vi "MF-101 Analog Output with diags and disk file.vi"() -> ()   [LabVIEW 8.6]
uses:
  <libdir>/resource/objmgr/ueidaq.rc
  <vilib>/Utility/file.llb/Write Delimited Spreadsheet (string).vi
  vi.lib/UeiDaq/UeiDaqConfigureTimingForSimpleIO.vi
  <vilib>/Utility/file.llb/Write Delimited Spreadsheet (DBL).vi
  vi.lib/UeiDaq/UeiDaqWriteOneScaledScan.vi
  vi.lib/UeiDaq/UeiDaqCreateAOSession.vi
  vi.lib/UeiDaq/UeiDaqCreateAOCurrentSession.vi
  vi.lib/UeiDaq/UeiDaqReadOneScaledScan.vi
panel:
  out "Diag Data":dbl[](array[numeric])
  in  "Diagnostic Resource":string
  in  "Maximum range":dbl
  in  "Minimum range":dbl
  in  "analog output":bool
  out "data points":i32
  in  "delta output":dbl format="%#_6f"
  in  "end  output":dbl
  in  "start output":dbl
  out "serial number":string
  out "name":string
  out "Waveform Chart":T1(graph)
  out "analog output(s)":dbl[](array[numeric])
  out "amplitude":dbl format="%#.6f"
  in  "Refresh rate (ms)":u32
  in  "stop":bool
  in  "Resource":string
  # "MF-101 Analog Output with Guardian diagnostics and disk file"
  # "Resource"
  # "Analog output settings"
  # "Device information"
  # "volts"
  # "amps"
  # "Analog Out diagnostics\n\n     Ch0 = temp_aout0\n     Ch1 = vsense_p_aout0\n     Ch2 = vsense_n_aout0\n     Ch3 = vdcp_p_aout0\n\n     Ch4 = temp_aout1\n     Ch5 = vsense_p_aout1\n     Ch6 = vsense_n_aout1\n     Ch7 = vdcp_p_aout1\n\npdna://192.168.100.2/dev0/Diag0"
  # "temp"
  # "vsense_p"
  # "vsense_n"
  # "vdcp_p"
  # "voltage ranges : +/-10V, +/-5V\ncurrent ranges : 0-20mA, 4-20mA, -1-22mA"
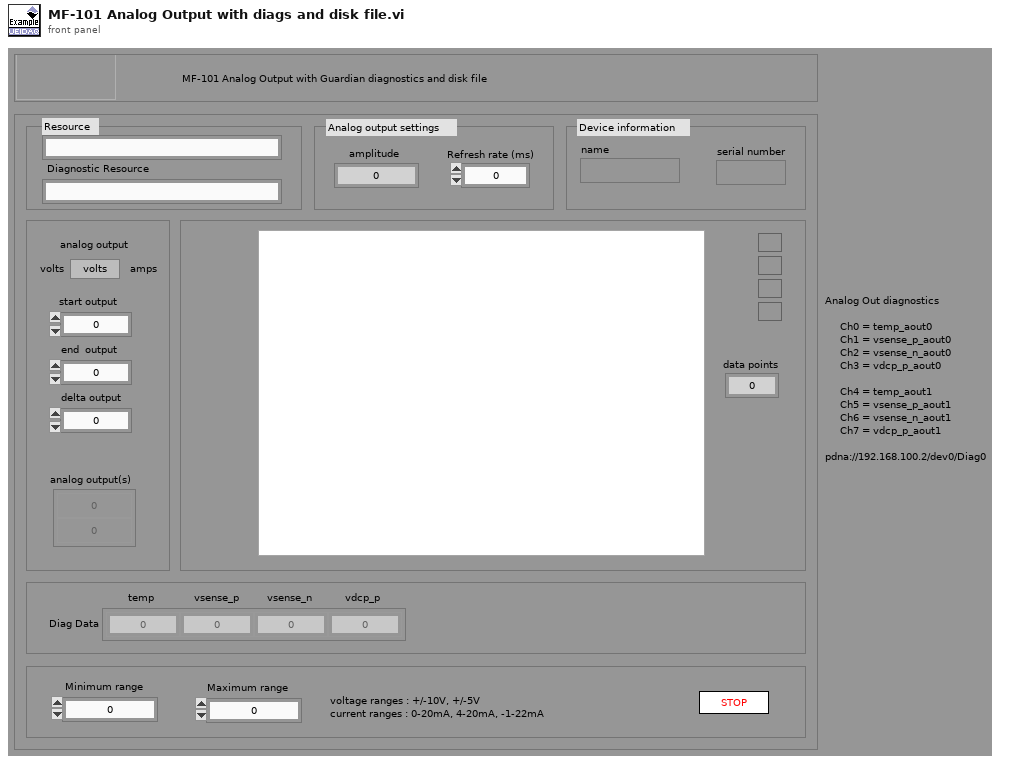
[diagram p1: front panel]
types:
  T1 = cluster{"[0]":dbl, "[1]":dbl, "[2]":dbl, "[3]":dbl, "[4]":dbl, "[5]":dbl, "[6]":dbl, "[7]":dbl, "[8]":dbl}
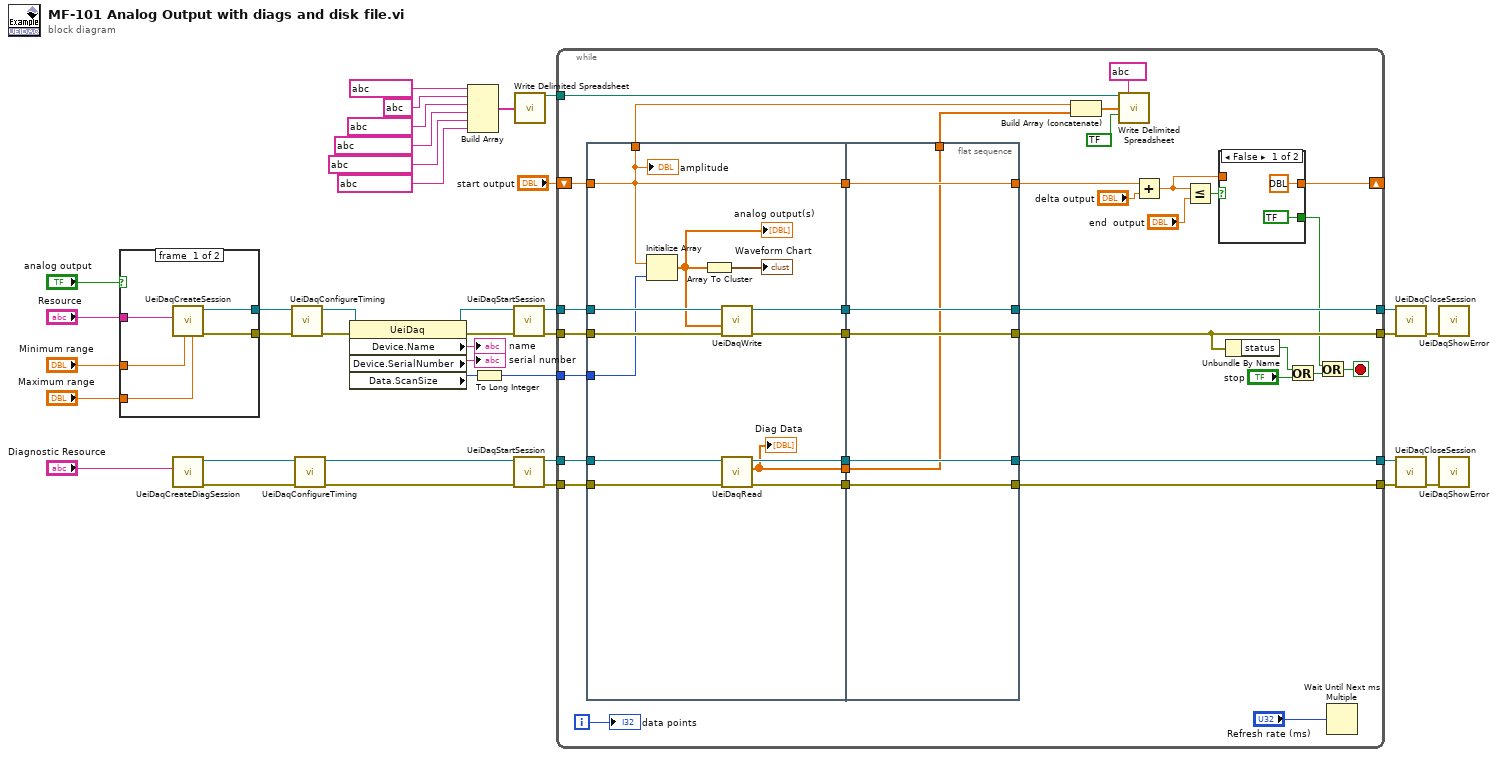
[diagram p0: block diagram]
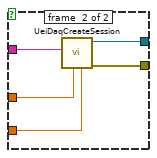
[diagram p2: hidden frame]
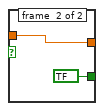
[diagram p3: hidden frame]
diagram:
  n1 = case shown="True" "analog output" {
    tunnel: "Resource" -> [w41 w48]
    tunnel: [w42 w47] -> w34
    tunnel: [w43 w46] -> w33
    tunnel: "Minimum range" -> [w40 w45]
    tunnel: "Maximum range" -> [w39 w44]
    frame #0 {
      n2 = call-poly "UeiDaqCreateSession.vi"("Maximum range"=w39, "Minimum range"=w40, "Resource"=w41) -> ("error out"=w43:errorcluster, "UeiDaq Refnum Out"=w42:refnum<k20>)  [unwired: 2 in, 5 out]
    }
    frame #1 {
      n3 = call-poly "UeiDaqCreateSession.vi"("Maximum range"=w44, "Minimum range"=w45, "Resource"=w48) -> ("error out"=w46:errorcluster, "UeiDaq Refnum Out"=w47:refnum<k20>)  [unwired: 2 in, 5 out]
    }
  }
  n4 = call "UeiDaqCreateDiagSession.vi"("Resource"="Diagnostic Resource") -> ("error out"=w6:errorcluster, "UeiDaq Refnum Out"=w7:refnum<k20>)  [unwired: 9 in]
  n5 = call-poly "UeiDaqConfigureTiming.vi"("error in (no error)"=w33, "UeiDaq Refnum In"=w34) -> ("error out"=w31:errorcluster, "UeiDaq Refnum Out"=w32:refnum<k20>)  [unwired: 8 out]
  n6 = call-poly "UeiDaqConfigureTiming.vi"("error in (no error)"=w6, "UeiDaq Refnum In"=w7) -> ("error out"=w14:errorcluster, "UeiDaq Refnum Out"=w15:refnum<k20>)  [unwired: 8 out]
  n7 = property class="UeiDaq"(reference=w32, error in=w31) -> (reference out=w17:refnum<k20>, error out=w19:errorcluster, "Device.Name"=→"name":string, "Device.SerialNumber"=→"serial number":string, "Data.ScanSize"=w29:u32)
  n8 = Build Array(string ?, string ?, string ? ("element"), string ? ("element"), string ? ("element"), string ? ("element")) -> (w22:string[])
  n9 = To Long Integer(number=w29) -> (32bit integer=w30:i32)
  n10 = call "UeiDaqStartSession.vi"("error in (no error)"=w19, "UeiDaq Refnum In"=w17) -> ("error out"=w18:errorcluster, "UeiDaq Refnum Out"=w16:refnum<k20>)  [unwired: 8 in]
  n11 = call "UeiDaqStartSession.vi"("error in (no error)"=w14, "UeiDaq Refnum In"=w15) -> ("error out"=w12:errorcluster, "UeiDaq Refnum Out"=w13:refnum<k20>)  [unwired: 8 in]
  n12 = call-poly <vilib>:"Write Delimited Spreadsheet.vi"("1D data"=w22) -> ("new file path (Not A Path if cancelled)"=w24:path)  [unwired: 13 in, 1 out]
  n13 = while {
    tunnel: w16 -> [w78]
    tunnel: w18 -> [w81]
    tunnel: [w80] -> w35
    tunnel: [w79] -> w36
    tunnel: w30 -> [w77]
    shift-right: [w71] -> _
    shift-left: "start output" -> [w67]
    tunnel: w24 -> [w60]
    tunnel: w13 -> [w56]
    tunnel: [w55] -> w10
    tunnel: w12 -> [w53]
    tunnel: [w52] -> w9
    i -> [w57]
    stop <- w68 stop-if-true
    n14 = flat-sequence {
      tunnel: w81 -> [w96]
      tunnel: w78 -> [w93]
      tunnel: w77 -> [w92]
      tunnel: w67 -> [w89]
      tunnel: [w95] -> w66
      tunnel: [w94] -> w65
      tunnel: [w89] -> w64
      tunnel: [w89] -> w58
      tunnel: w56 -> [w88]
      tunnel: [w87] -> w54
      tunnel: w53 -> [w86]
      tunnel: [w85] -> w51
      tunnel: [w84] -> w50
      tunnel: [w100] -> w59
      tunnel: [w101] -> w79
      tunnel: [w102] -> w80
      tunnel: w66 -> [w102]
      tunnel: w65 -> [w101]
      tunnel: w64 -> [w100]
      tunnel: [w99] -> w55
      tunnel: w54 -> [w99]
      tunnel: [w98] -> w52
      tunnel: w51 -> [w98]
      tunnel: w50 -> [w97]
      tunnel: [w97] -> w49
      frame #0 {
        n15 = Initialize Array(w89, w92) -> (w91:dbl[])
        "analog output(s)" <- w91
        n16 = Array To Cluster(array=w91) -> (cluster=→"Waveform Chart":T1)
        n17 = call-poly "UeiDaqWrite.vi"("error in (no error)"=w96, "Scaled Data"=w91, "UeiDaq Refnum In"=w93) -> ("error out"=w95:errorcluster, "UeiDaq Refnum Out"=w94:refnum<k20>)  [unwired: 1 in, 6 out]
        n18 = call-poly "UeiDaqRead.vi"("error in (no error)"=w86, "UeiDaq Refnum In"=w88) -> ("error out"=w85:errorcluster, "Scaled Data"=w84:dbl[], "UeiDaq Refnum Out"=w87:refnum<k20>)  [unwired: 7 in]
        "Diag Data" <- w84
        "amplitude" <- w89
      }
      frame #1 {
      }
    }
    n19 = Build Array (concatenate)(w58, w49) -> (w63:dbl[])
    n20 = call-poly <vilib>:"Write Delimited Spreadsheet.vi"("file path (dialog if empty)"=w60, "format (%.3f)"=string ?, "1D data"=w63, "append to file? (new file:F)"=bool ?) -> ()  [unwired: 10 in, 2 out]
    n21 = Add(x=w59, y="delta output") -> (x+y=w75:dbl)
    n22 = Less Or Equal?(x=w75, y="end  output") -> (x <= y?=w74:bool)
    n23 = case shown="False" w74 {
      tunnel: w75 -> [_ w106]
      tunnel: [dbl ? w106] -> w71
      tunnel: [bool ? bool ?] -> w69
      frame #0 {
      }
      frame #1 {
      }
    }
    n24 = Unbundle By Name(w80) -> ("status"=w83:bool)
    n25 = Or(x=w83, y="stop") -> (x .or. y?=w70:bool)
    n26 = Or(x=w69, y=w70) -> (x .or. y?=w68:bool)
    n27 = Wait Until Next ms Multiple(millisecond multiple="Refresh rate (ms)") -> ()  [unwired: 1 out]
    "data points" <- w57
  }
  n28 = call "UeiDaqCloseSession.vi"("error in (no error)"=w35, "UeiDaq Refnum In"=w36) -> ("error out"=w38:errorcluster)  [unwired: 1 in, 8 out]
  n29 = call "UeiDaqCloseSession.vi"("error in (no error)"=w9, "UeiDaq Refnum In"=w10) -> ("error out"=w11:errorcluster)  [unwired: 1 in, 8 out]
  n30 = call "UeiDaqShowError.vi"("error in (no error)"=w38) -> ()  [unwired: 2 in, 9 out]
  n31 = call "UeiDaqShowError.vi"("error in (no error)"=w11) -> ()  [unwired: 2 in, 9 out]
